vi "control_esp.vi"() -> ()   [LabVIEW 2018]
uses:
  <vilib>/Utility/file.llb/Write Delimited Spreadsheet (I64).vi
panel:
  out "String":string
  in  "Right":bool
  in  "Forward":bool
  in  "Left":bool
  in  "Backward":bool
  in  "stop":bool
  in  "Port":u16=1234
  in  "string 12":string
  in  "string 11":string
  in  "string 10":string="168"
  in  "string 9":string="192"
  in  "Cluster":cluster{"type":string, "content":string}={"type"="get_binary_image", "content"="image"}
  out "error out":errorcluster={"status"=TRUE, "code"=-375003, "source"="Unflatten From JSON in control_esp.vi"}
  out "new picture":picture
  in  "header size":i8=10
  in  "Port 2":u16=1234
  in  "string 8":string="9"
  in  "string 7":string="1"
  in  "string 6":string="168"
  in  "string 5":string="192"
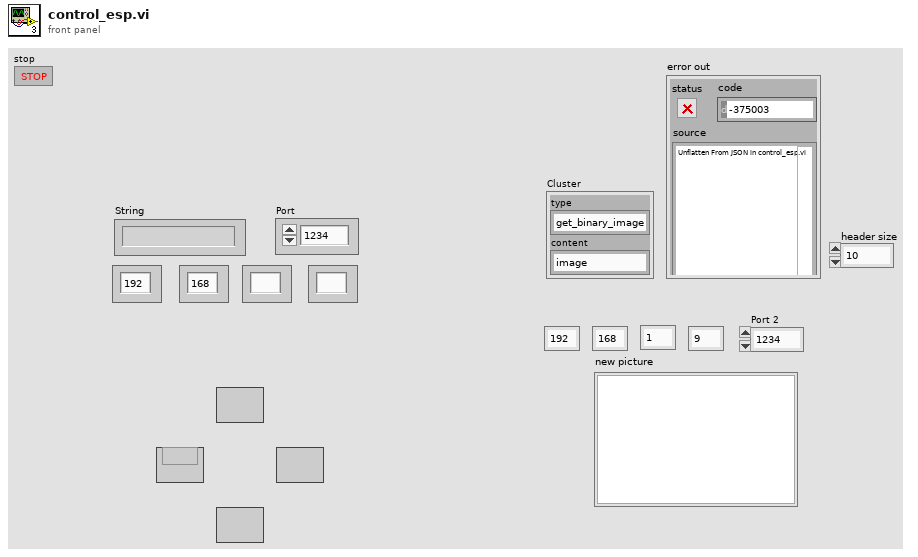
[diagram p1: front panel]
types:
  T1 = typedef "imagedata.ctl" = cluster{"image type":i32, "image depth":i32, "image":u8[], "mask":u8[], "colors":u32[], "Rectangle":cluster{"left":i16, "top":i16, "right":i16, "bottom":i16}}
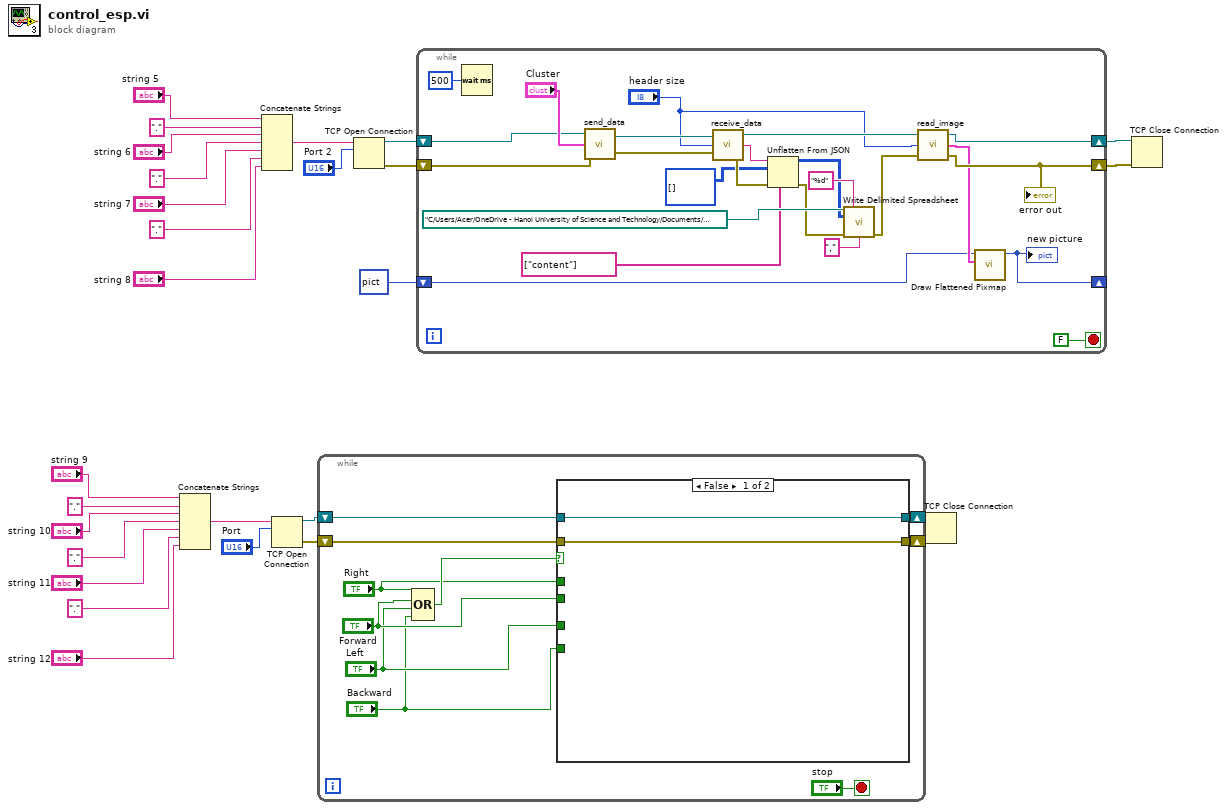
[diagram p0: block diagram]
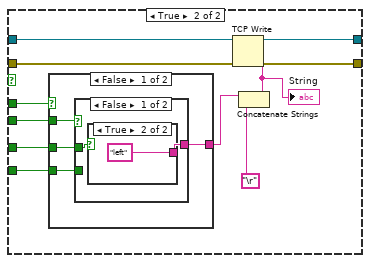
[diagram p2: hidden frame]
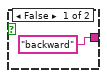
[diagram p3: hidden frame]
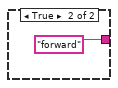
[diagram p4: hidden frame]
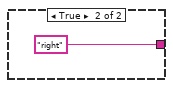
[diagram p5: hidden frame]
diagram:
  n1 = Concatenate Strings("string 9", ".", "string 10", ".", "string 11", ".", "string 12") -> (w6:string)
  n2 = Concatenate Strings("string 5", ".", "string 6", ".", "string 7", ".", "string 8") -> (w20:string)
  n3 = TCP Open Connection(address=w6, remote port or service name="Port") -> (connection ID=w5:refnum<k5>, error out=w2:errorcluster)  [unwired: 3 in]
  n4 = while {
    shift-right: [w36] -> w4
    shift-left: w5 -> [w37]
    shift-right: [w35] -> w3
    shift-left: w2 -> [w34]
    stop <- "stop" stop-if-true
    n5 = Compound Arithmetic op=OR("Right", "Forward", "Left", "Backward") -> (w33:bool)
    n6 = case shown="False" w33 {
      tunnel: w37 -> [w39 w50]
      tunnel: [w39 w49] -> w36
      tunnel: [w38 w48] -> w35
      tunnel: w34 -> [w38 w47]
      tunnel: "Right" -> [_ w45]
      tunnel: "Forward" -> [_ w43]
      tunnel: "Left" -> [_ w42]
      tunnel: "Backward" -> [_ w41]
      frame False {
      }
      frame True {
        n7 = case shown="False" w45 {
          tunnel: [w53 "right"] -> w44
          tunnel: w43 -> [w54 _]
          tunnel: w42 -> [w52 _]
          tunnel: w41 -> [w51 _]
          frame False {
            n8 = case shown="False" w54 {
              tunnel: [w55 "forward"] -> w53
              tunnel: w52 -> [w56 _]
              tunnel: w51 -> [_ _]
              frame False {
                n9 = case shown="True" w56 {
                  tunnel: ["backward" "left"] -> w55
                  frame False {
                  }
                  frame True {
                  }
                }
              }
              frame True {
              }
            }
          }
          frame True {
          }
        }
        n10 = Concatenate Strings(w44, "\r") -> (w40:string)
        "String" <- w40
        n11 = TCP Write(connection ID=w50, data in=w40, error in (no error)=w47) -> (connection ID out=w49:refnum<k5>, error out=w48:errorcluster)  [unwired: 1 in, 1 out]
      }
    }
  }
  n12 = TCP Open Connection(address=w20, remote port or service name="Port 2") -> (connection ID=w18:refnum<k5>, error out=w17:errorcluster)  [unwired: 3 in]
  n13 = while {
    shift-right: [w67] -> w16
    shift-left: w18 -> [w83]
    shift-right: [w66] -> w15
    shift-left: w17 -> [w82]
    shift-right: [w61] -> _
    shift-left: picture data[5B] ("picture") -> [w62]
    stop <- FALSE stop-if-true
    n14 = Wait (ms)(milliseconds to wait=u32 500) -> ()  [unwired: 1 out]
    n15 = call "send_data.vi"("error in"=w82, "Cluster"="Cluster", "connection ID"=w83) -> ("error out"=w80:errorcluster, "connection ID out"=w81:refnum<k5>)  [unwired: 1 in]
    n16 = call "receive_data.vi"("error in"=w80, "header size"="header size", "connection ID"=w81) -> ("error out"=w77:errorcluster, "data out"=w78:string, "connection ID out"=w70:refnum<k5>)
    n17 = Unflatten From JSON(path=string[] ["content"], JSON string=w78, type and defaults=i16[][] [], error in (no error)=w77) -> (value=w71:i16[][], error out=w76:errorcluster)  [unwired: 3 in]
    n18 = call-poly <vilib>:"Write Delimited Spreadsheet.vi"("file path (dialog if empty)"=path "C:/Users/Acer/OneDrive - Hanoi University of Science and Technology/Documents/LabViewProject/Project/labview/data.csv", "format (%d)"="%d" ("format (%.3f)"), "2D data"=w71, "error in (no error)"=w76, "delimiter (\\t)"="," ("delimiter (\\t)")) -> ("error out"=w68:errorcluster)  [unwired: 9 in, 1 out]
    n19 = call "read_image.vi"("error in"=w68, "header size"="header size", "connection ID"=w70) -> ("error out"=w66:errorcluster, "image data"=w65:T1, "connection ID out"=w67:refnum<k5>)
    "error out" <- w66
    n20 = call <vilib>:"Draw Flattened Pixmap.vi"("image data"=w65, "picture"=w62) -> ("new picture"=w61:picture)  [unwired: 7 in]
    "new picture" <- w61
  }
  n21 = TCP Close Connection(connection ID=w4, error in (no error)=w3) -> ()  [unwired: 1 in, 2 out]
  n22 = TCP Close Connection(connection ID=w16, error in (no error)=w15) -> ()  [unwired: 1 in, 2 out]
